vi "Write Upper Limit_Limit.vi"(8 "error in (no error)":errorcluster, 10 "Upper Limit/Limit":dbl, 11 "Numeric Limit Compare Config in":refnum<class "Numeric Limit Compare Config.lvclass">) -> (0 "error out":errorcluster, 3 "Numeric Limit Compare Config out":refnum<class "Numeric Limit Compare Config.lvclass">)   [LabVIEW 2015, in "Numeric Limit Compare Config.lvclass"]
uses:
  Numeric Limit Compare Config.lvclass
  Numeric Limit Compare Config.lvclass/Numeric Limit Compare Config.ctl
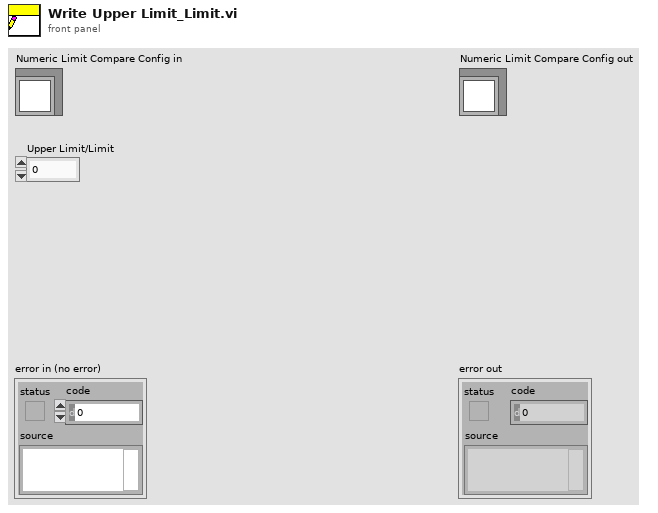
[diagram p1: front panel]
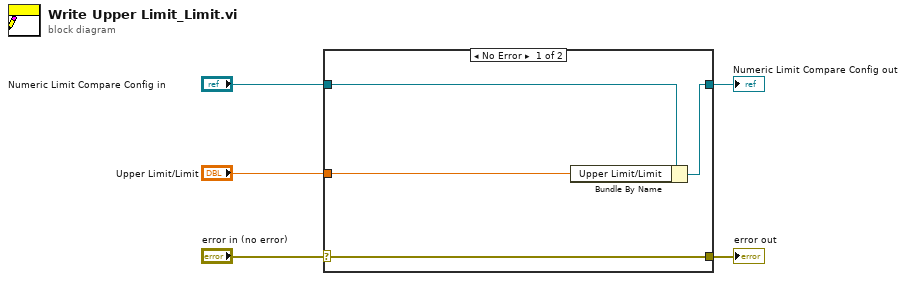
[diagram p0: block diagram]
diagram:
  n1 = case shown="No Error" "error in (no error)" {
    selector: "error in (no error)" -> [w9 w10]
    tunnel: [w9 w10] -> w4
    tunnel: [w7 w11] -> w2
    tunnel: "Numeric Limit Compare Config in" -> [w8 w11]
    tunnel: "Upper Limit/Limit" -> [w6 _]
    frame No Error {
      n2 = Bundle By Name(cluster=w8, "Upper Limit/Limit"=w6) -> (w7:refnum<class "Numeric Limit Compare Config.lvclass">)
    }
    frame Error {
    }
  }
  "error out" <- w4
  "Numeric Limit Compare Config out" <- w2
